vi "T7_Read_Float_Registers.vi"(6 "Num Registers":u16=2, 8 "error in (no error)":errorcluster, 9 "FirstChannel":u16, 10 "Remote Port":u16=502, 11 "Remote IP Address":string="192.168.1.15") -> (0 "error out":errorcluster, 1 "ReadAt":timestamp, 2 "LastValue":dbl, 3 "Array":dbl[](array[numeric]))   [LabVIEW 2014]
uses:
  Serial Link Layer/NI_Modbus_Cleaned/NI Modbus121Clean.llb/MB Ethernet Master Query Read Input Registers (poly).vi
panel:
  out "Starting Address":u16
  out "Results (binary)":u16[](array[numeric])
  # "TCP Parameters"
  # "Slave Read-only Registers"
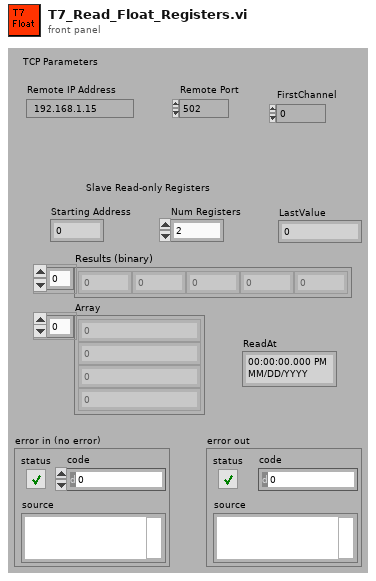
[diagram p1: front panel]
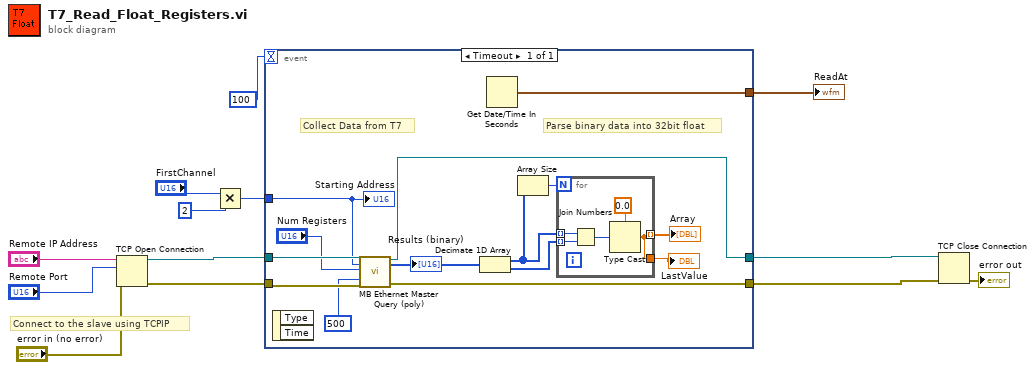
[diagram p0: block diagram]
diagram:
  # "Connect to the slave using TCPIP"
  n1 = TCP Open Connection(address="Remote IP Address", remote port or service name="Remote Port", error in (no error)="error in (no error)") -> (connection ID=w11:refnum<k5>, error out=w10:errorcluster)  [unwired: 2 in]
  n2 = Multiply(x="FirstChannel", y=u16 2) -> (x*y=w1:u16)
  n3 = event shown="[0] Timeout" {
    selector: _ -> [_]
    dyn-events: _ -> [_]
    timeout: 100 -> [_]
    tunnel: [w23] -> w9
    tunnel: w11 -> [w27]
    tunnel: w10 -> [w26]
    tunnel: [w24] -> w8
    tunnel: [w15] -> w4
    tunnel: w1 -> [w14]
    event Timeout {
      # "Parse binary data into 32bit float"
      # "Collect Data from T7"
      n4 = event-data() -> ()  [unwired: 3 out]
      n5 = call-poly "MB Ethernet Master Query (poly).vi"("TCP Connection Refnum in"=w27, "Starting Address"=w14, "Quantity"="Num Registers", "Timeout"=500, "error in"=w26) -> ("TCP Connection Refnum (dup)"=w24:refnum<k5>, "Input Registers"=w22:u16[], "error out"=w23:errorcluster)  [unwired: 11 in, 1 out]
      "Results (binary)" <- w22
      n6 = Decimate 1D Array(w22) -> (w20:u16[], w19:u16[])
      n7 = Get Date/Time In Seconds() -> (seconds since 1Jan1904=w15:timestamp)
      n8 = Array Size(array=w20) -> (size(s)=w21:i32)
      n9 = for {
        N: w21 -> [_]
        tunnel: w20 -> [w31] mode=indexing
        tunnel: w19 -> [w32] mode=indexing
        tunnel: [w28] -> w18 mode=indexing
        tunnel: [w28] -> w17
        n10 = Join Numbers(hi=w31, lo=w32) -> ((hi.lo)=w30:u32)
        n11 = Type Cast(type=sgl 0.0, x=w30) -> (*(type *) &x=w28:sgl)
      }
      "Array" <- w18
      "LastValue" <- w17
      "Starting Address" <- w14
    }
  }
  "ReadAt" <- w4
  n12 = TCP Close Connection(connection ID=w8, error in (no error)=w9) -> (error out=→"error out":errorcluster)  [unwired: 2 out]
